vi "LJM_eWriteAddresses.vi"(0 "Handle In":i32, 1 "NumFrames (Auto-Detect)":i32=-1, 5 "aAddresses":i32[](array[numeric]), 7 "aTypes":i32[](array[numeric]), 9 "aValues":dbl[](array[numeric]) format="%.2f", 11 "error in":errorcluster) -> (4 "Handle Out":i32, 14 "ErrorAddress":i32, 15 "error out":errorcluster)   [LabVIEW 2024]
uses:
  labjackm.dll
panel:
  # "1/20/2015:  Default value of NumFrames changed to -1 which\nequates to Auto-Detect.  If NumFrames = -1, then the NumFrames\ncontrol is ignored and the size of aNames/aAddresses is used to\ndetermine how many frames there are."
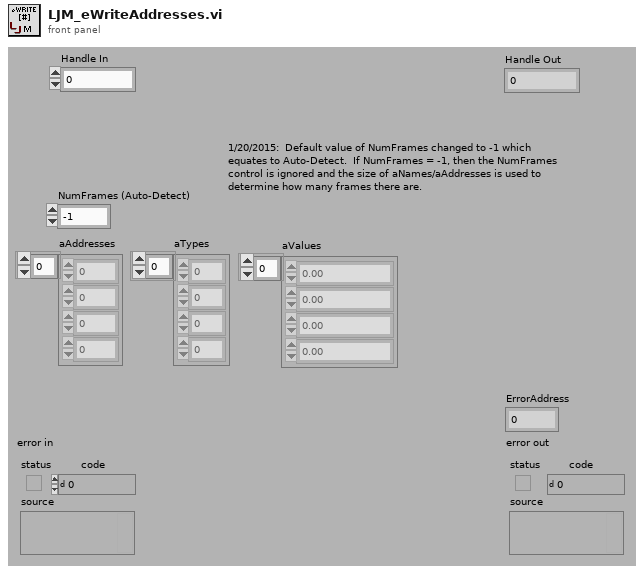
[diagram p1: front panel]
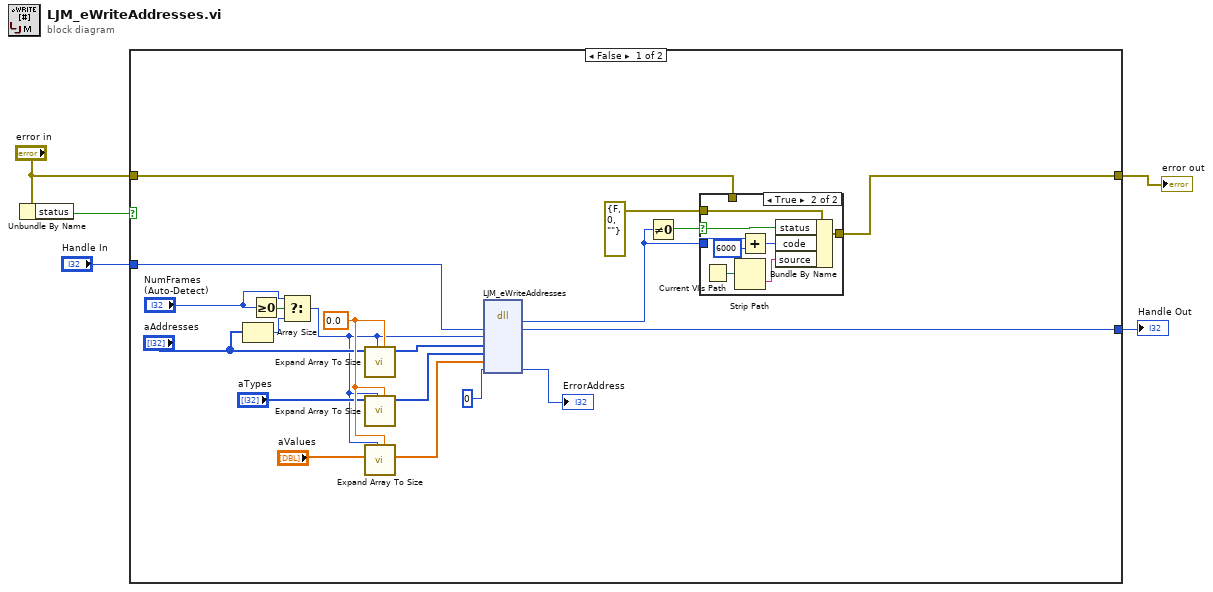
[diagram p0: block diagram]
diagram:
  n1 = Unbundle By Name("error in") -> ("status"=w5:bool)
  n2 = case shown="False" w5 {
    tunnel: "error in" -> [w22 w36]
    tunnel: [w21 w36] -> w3
    tunnel: "Handle In" -> [w12 w35]
    tunnel: [w11 w35] -> w1
    frame False {
      w19 = 0.0 ("Default Value")
      n3 = Array Size(array="aAddresses") -> (size(s)=w10:i32)
      n4 = Greater Or Equal To 0?(x="NumFrames (Auto-Detect)") -> (x >= 0?=w9:bool)
      n5 = Select(t="NumFrames (Auto-Detect)", s=w9, f=w10) -> (s? t:f=w6:i32)
      n6 = call "Expand Array To Size.vi"("Default Value"=w19, "# Elements"=w6, "I32 Array In"="aAddresses") -> ("I32 Array Out"=w20:i32[])  [unwired: 4 in, 4 out]
      n7 = call "Expand Array To Size.vi"("Default Value"=w19, "# Elements"=w6, "I32 Array In"="aTypes") -> ("I32 Array Out"=w17:i32[])  [unwired: 4 in, 4 out]
      n8 = call "Expand Array To Size.vi"("Default Value"=w19, "# Elements"=w6, "DBL Array In"="aValues") -> ("DBL Array Out"=w16:dbl[])  [unwired: 4 in, 4 out]
      n9 = dll-call lib="labjackm.dll" fn="LJM_eWriteAddresses"("Handle"=w12, "NumFrames"=w6, "aAddresses"=w20, "aTypes"=w17, "aValues"=w16, "ErrorFrame"=u32 0) -> (w25:i32, "Handle"=w11:i32, "ErrorFrame"=→"ErrorAddress":i32)  [unwired: 7 in, 2 out]
      n10 = Not Equal To 0?(x=w25) -> (x != 0?=w24:bool)
      n11 = case shown="True" w24 {
        selector: w24 -> [_ w33]
        tunnel: [w26 w34] -> w21
        tunnel: errorcluster {"status"=FALSE, "code"=0, "source"=""} ("error IO") -> [_ w32]
        tunnel: w25 -> [_ w28]
        tunnel: w22 -> [w26 _]
        frame False {
        }
        frame True {
          n12 = Current VI's Path() -> (path=w30:path)
          n13 = Strip Path(path=w30) -> (name=w31:string)  [unwired: 1 out]
          n14 = Add(x=w28, y=6000) -> (x+y=w29:i32)
          n15 = Bundle By Name(cluster=w32, "status"=w33, "code"=w29, "source"=w31) -> (w34:errorcluster)
        }
      }
    }
    frame True {
    }
  }
  "error out" <- w3
  "Handle Out" <- w1
